vi "Spara List or All.vi"(11 "S## Type":string) -> (3 "S## List or All?":bool)   [LabVIEW 2011]
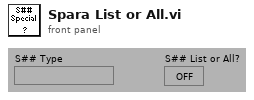
[diagram p1: front panel]
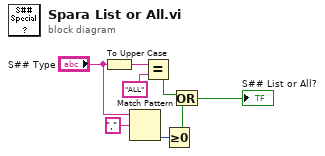
[diagram p0: block diagram]
diagram:
  n1 = To Upper Case(1:"S## Type") -> (0:w2:string)
  n2 = Match Pattern(string="S## Type", regular expression=",") -> (offset past match=w7:i32)  [unwired: 4 out]
  n3 = Equal?(x=w2, y="ALL") -> (x = y?=w4:bool)
  n4 = Greater Or Equal To 0?(x=w7) -> (x >= 0?=w8:bool)
  n5 = Or(x=w4, y=w8) -> (x .or. y?=→"S## List or All?":bool)
